vi "MB_TCP_X.vi"(6 "N":i32, 9 "timeouts":T1={"conn_timeout"=1000, "reconn_timeout"=3000, "N attempt max"=3, "t_reset_TTL"=120000, "write_timeout"=10, "read_timeout"=500, "period"=100} {"t_reset_TTL" min=10 max=240000 step=1; "period" min=10 max=100000 step=1; "read_timeout" min=10 max=60000 step=1; "write_timeout" min=1 max=60000 step=1; "N attempt max" min=1 max=5 step=1; "reconn_timeout" min=10 max=240000 step=1; "conn_timeout" min=10 max=240000}, 10 "write enable":bool=TRUE, 11 "stop":bool) -> (0 "error out":errorcluster, 2 "errors":u32, 3 "Z3":u32)   [LabVIEW 2019, in "MB_TCP1.lvlib"]
uses:
  MB_TCP1.lvlib
  Userlib.lvlib
  NI_modbus_upd/NI_modbus_upd.lvlib
  NI_modbus_upd.llb/MB Modbus Command.ctl
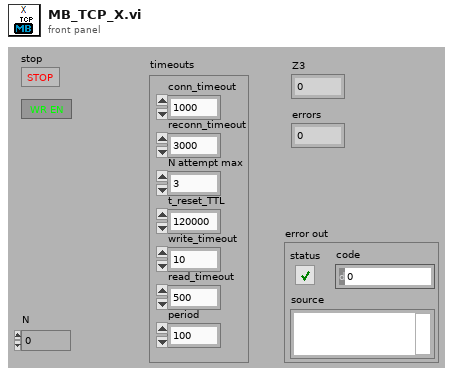
[diagram p1: front panel]
types:
  T1 = cluster{"conn_timeout":i32, "reconn_timeout":u32, "N attempt max":i32, "t_reset_TTL":u32, "write_timeout":i32, "read_timeout":i32, "period":u32}
  T2 = enum16{"Init", "Read", "Read inputs", "Read outputs", "Write", "Write inputs"}
  T3 = enum16{"DI", "DO to write", "DO", "AI", "AO to write", "AO", "DI AI", "DI AO", "DO AI", "DO AO"}
  T4 = enum16{"Start", "Connect", "Write enable", "IP address", "Errors"}
  T5 = typedef "MB Modbus Command.ctl" = cluster{"Function Code":u8, "Starting Address":u16, "Quantity":u16, "Data":u16[], "Discrete":bool[]}
  T6 = cluster{"Transaction ID":u16, "Protocol ID":u16, "Length":u16, "Unit ID":u8}
  T7 = cluster{"Remote IP Address":string, "Remote Port":u16}
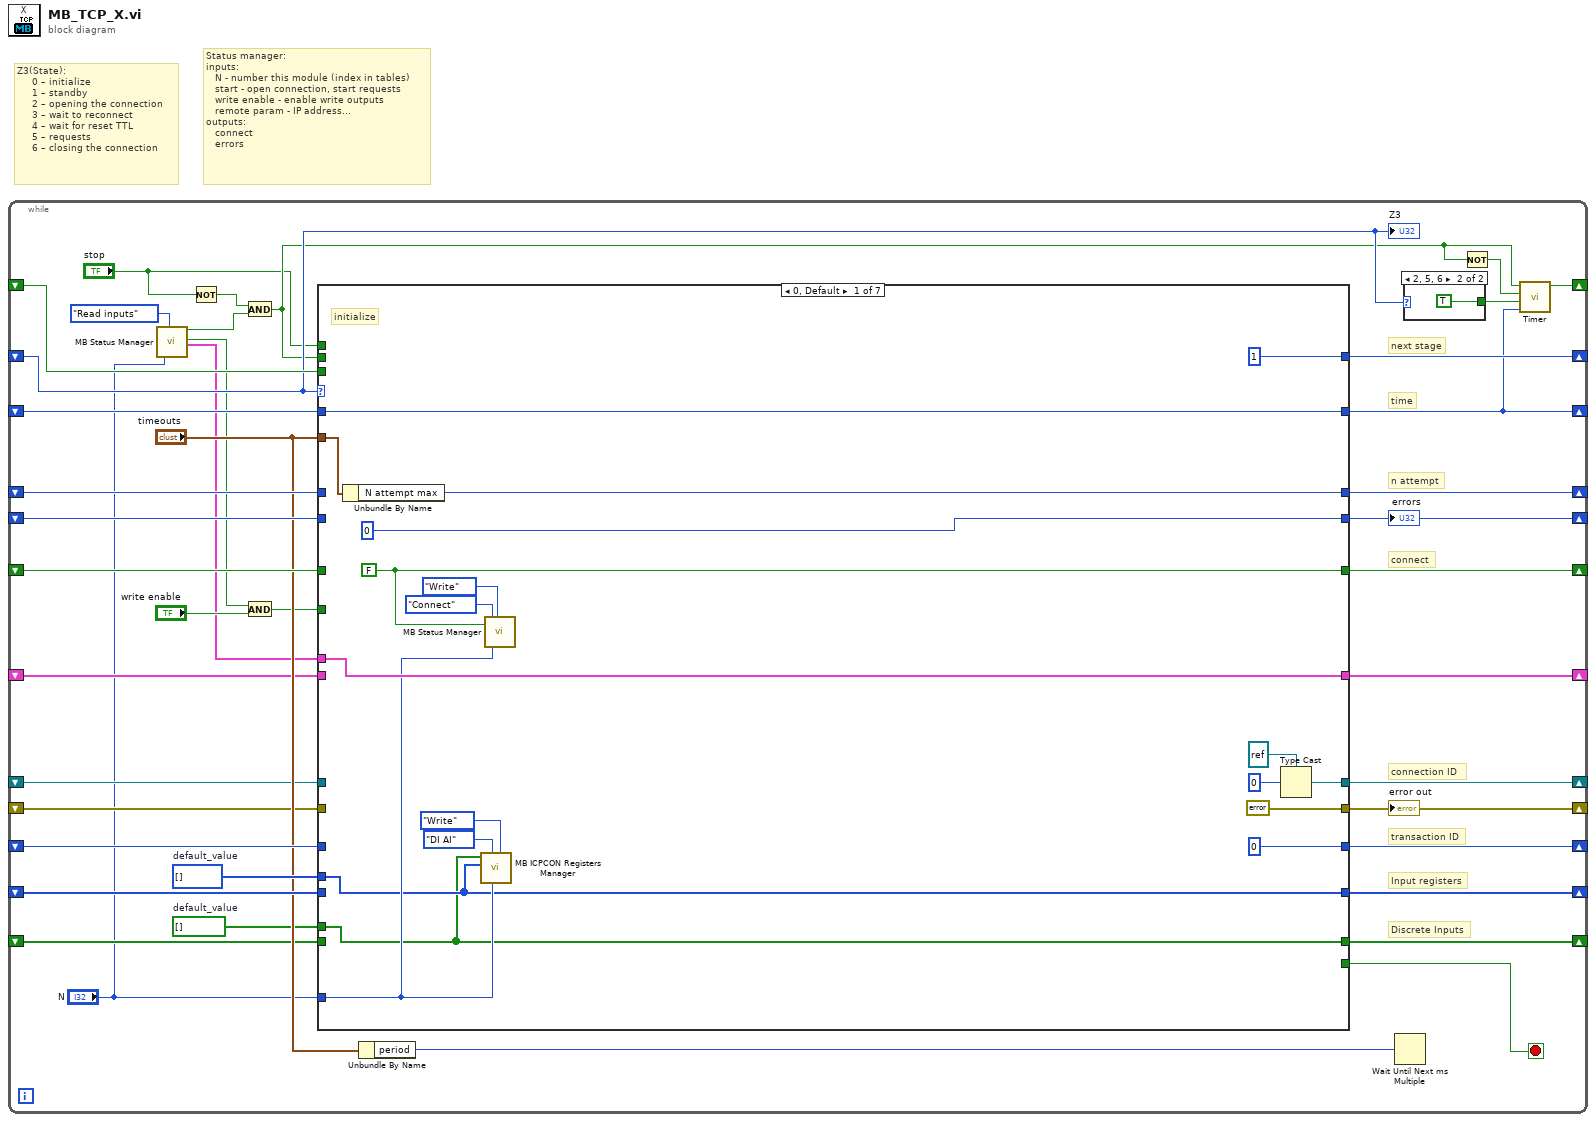
[diagram p0: block diagram]
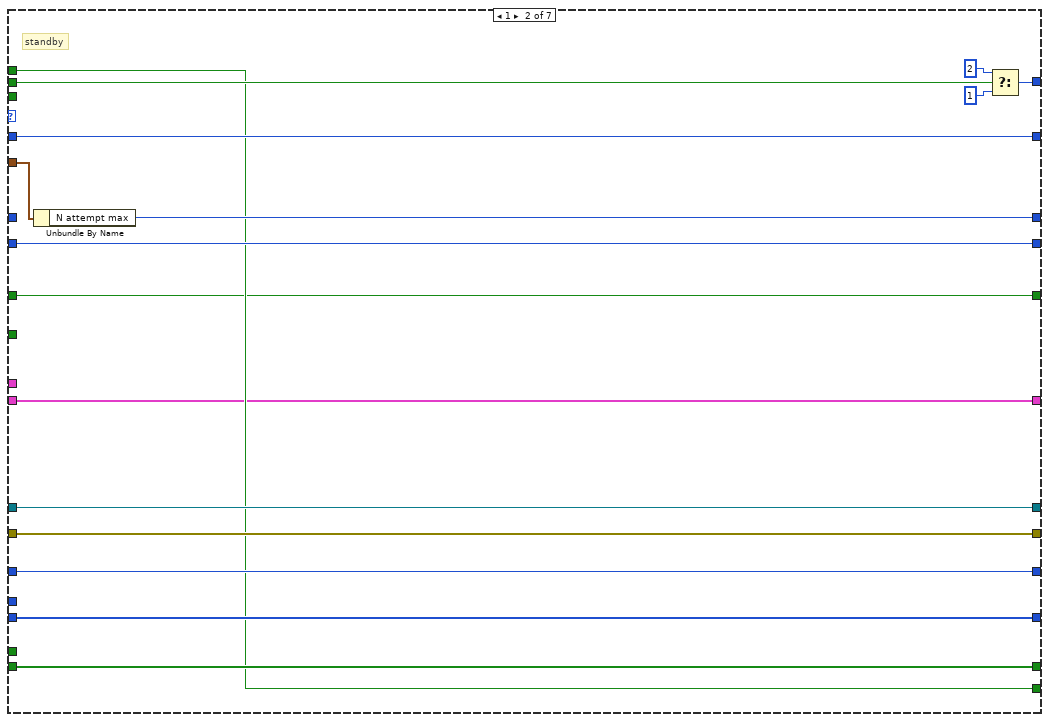
[diagram p2: hidden frame]
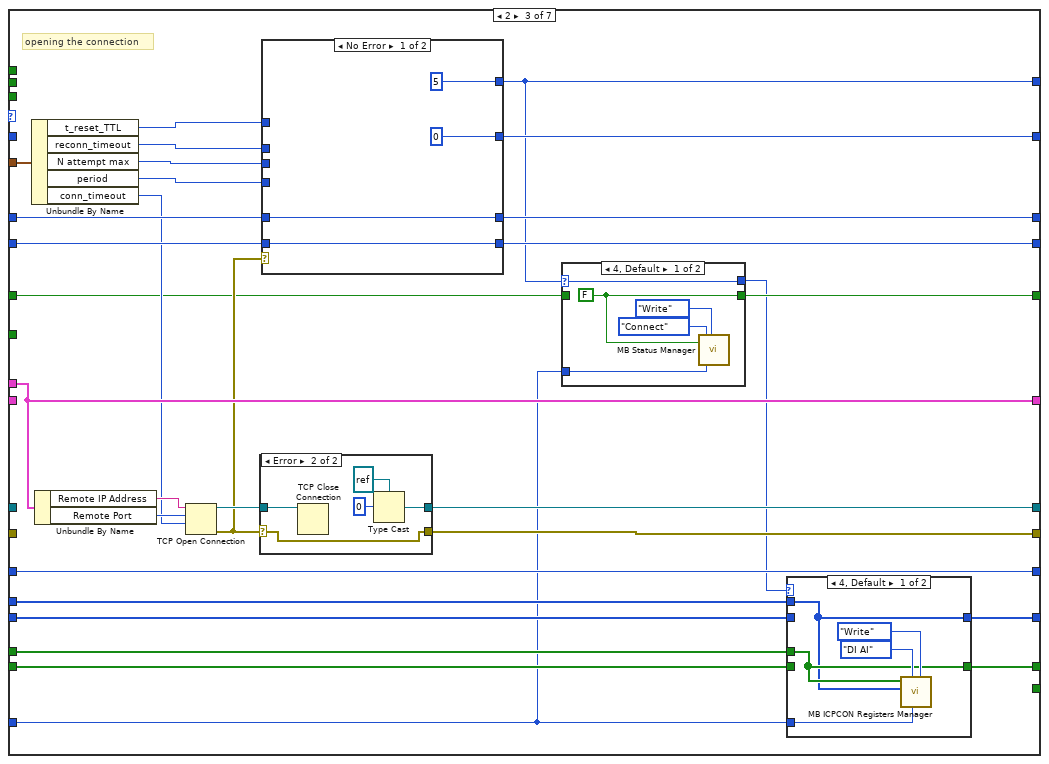
[diagram p3: hidden frame]
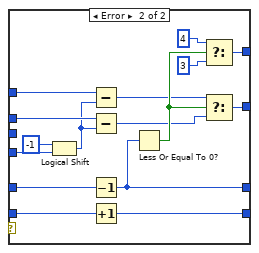
[diagram p7: hidden frame]
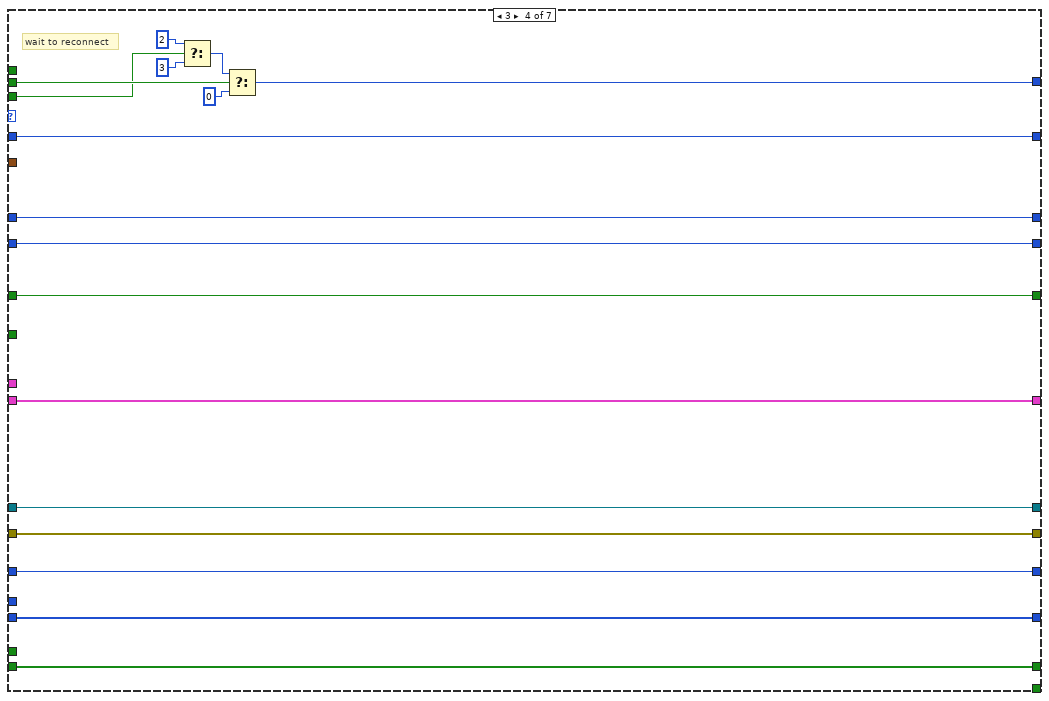
[diagram p8: hidden frame]
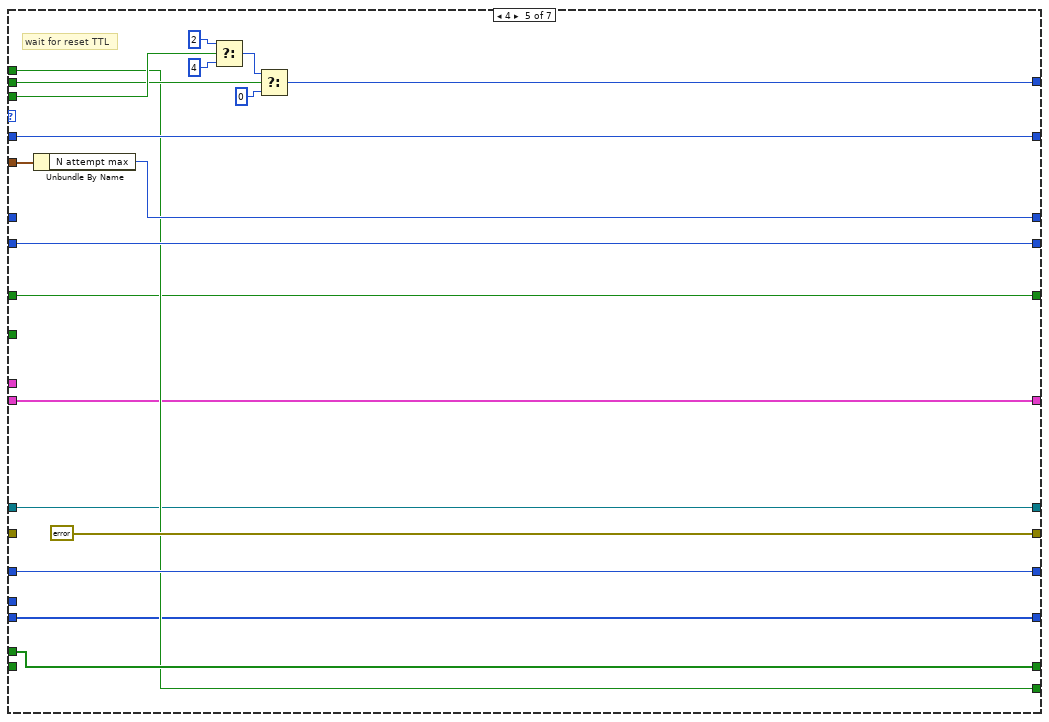
[diagram p9: hidden frame]
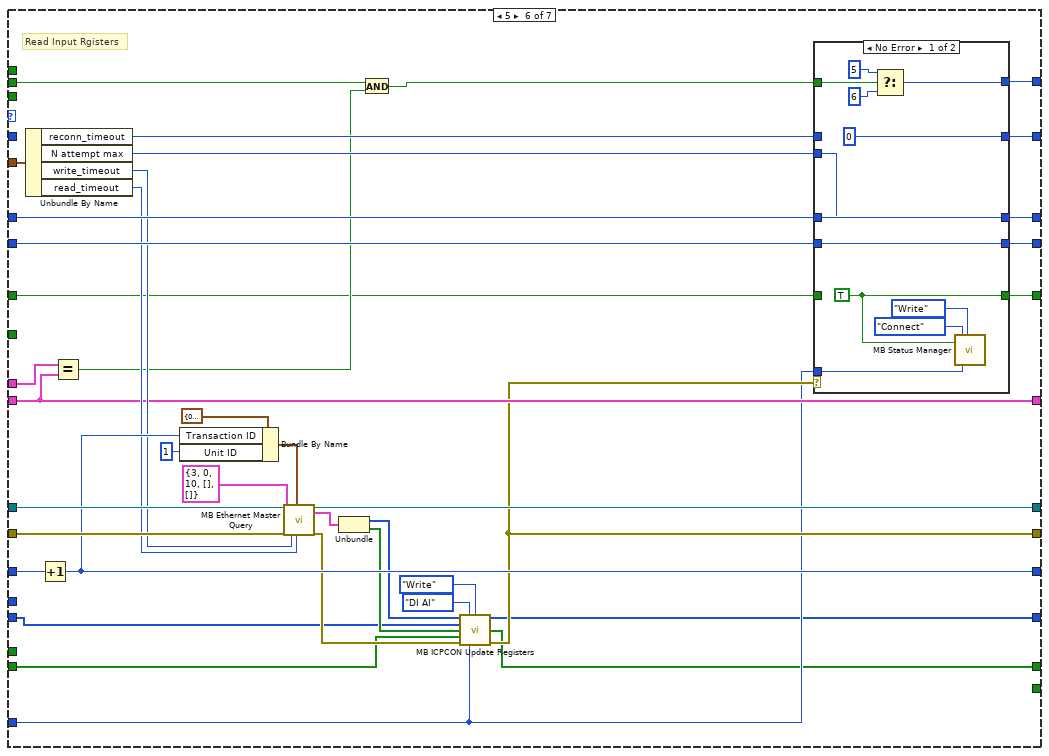
[diagram p10: hidden frame]
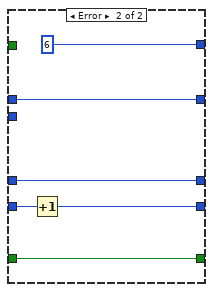
[diagram p11: hidden frame]
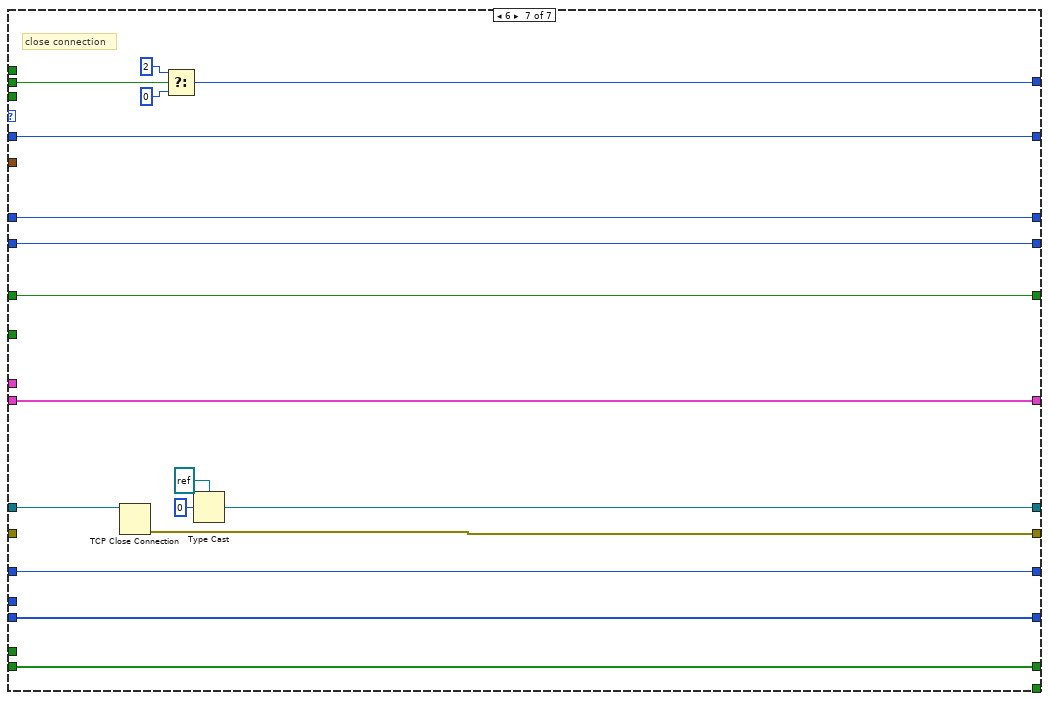
[diagram p12: hidden frame]
diagram:
  # "Status manager:\ninputs:\n   N - number this module (index in tables)\n   start - open connection, start requests\n   write enable - enable write outputs\n   remote param - IP address...\noutputs:\n   connect\n   errors"
  # "Z3(State):\n     0 – initialize \n     1 – standby\n     2 – opening the connection\n     3 – wait to reconnect\n     4 – wait for reset TTL\n     5 – requests\n     6 – closing the connection"
  n1 = while {
    shift-right: [w18] -> _
    shift-left: _ -> [w14]
    shift-right: [w17] -> _
    shift-left: _ -> [w40]
    shift-right: [w39] -> _
    shift-left: _ -> [w37]
    shift-right: [w38] -> _
    shift-left: _ -> [w36]
    shift-right: [w35] -> _
    shift-left: _ -> [w34]
    shift-right: [w33] -> _
    shift-left: _ -> [w19]
    shift-right: [w32] -> _
    shift-left: _ -> [w20]
    shift-right: [w31] -> _
    shift-left: _ -> [w30]
    shift-right: [w29] -> _
    shift-left: _ -> [w28]
    shift-right: [w22] -> _
    shift-left: _ -> [w21]
    shift-right: [w16] -> _
    shift-left: _ -> [w15]
    shift-right: [w7] -> _
    shift-left: _ -> [w6]
    stop <- w10 stop-if-true
    w23 = bool[] []  # default_value
    w27 = u16[] []  # default_value
    # "Discrete Inputs"
    # "Input registers"
    # "connect"
    # "connection ID"
    # "transaction ID"
    # "n attempt"
    # "time"
    # "next stage"
    n2 = call "MB Status Manager.vi"("N"="N", "Function"=T2."Read inputs") -> ("start"=w5:bool, "write enable"=w4:bool, "Remote Param"=w3:T7)  [unwired: 12 in, 3 out]
    n3 = Not(x="stop") -> (.not. x?=w12:bool)
    n4 = And(x=w12, y=w5) -> (x .and. y?=w13:bool)
    n5 = And(x=w4, y="write enable") -> (x .and. y?=w9:bool)
    n6 = case shown="0, Default" w14 {
      tunnel: [w58 w67 w84 w162 w168 w210 w253] -> w33
      tunnel: [errorcluster {"status"=FALSE, "code"=0, "source"=""} ("error out") w66 w82 w161 errorcluster {"status"=FALSE, "code"=0, "source"=""} ("error out") w193 w254] -> w32
      tunnel: w19 -> [_ w67 _ w162 w168 w212 w250]
      tunnel: w20 -> [_ w66 _ w161 _ w211 _]
      tunnel: [w47 w62 w80 w150 w167 w195 w241] -> w35
      tunnel: w34 -> [_ w62 w81 w150 w167 w196 w241]
      tunnel: w3 -> [w50 _ w87 _ _ w202 _]
      tunnel: [w45 w68 w92 w149 w166 w189 w240] -> w29
      tunnel: w28 -> [_ w68 w93 w149 w166 w184 w240]
      tunnel: w30 -> [_ w76 w106 w164 w183 w221 w255]
      tunnel: [u16 0 ("x") w76 w106 w164 w183 w206 w255] -> w31
      tunnel: [w52 w72 w101 w163 w179 w219 w247] -> w39
      tunnel: w37 -> [_ _ w102 w163 _ w219 w247]
      tunnel: [u32 0 ("N attempt max") w75 w104 w160 w182 w218 w252] -> w38
      tunnel: w36 -> [_ w75 w105 w160 w182 w217 w252]
      tunnel: [w54 w74 w98 w159 w181 w214 w251] -> w17
      tunnel: w40 -> [w54 w74 _ w159 w181 _ w251]
      tunnel: "timeouts" -> [w53 w73 w103 _ w180 w220 _]
      tunnel: w13 -> [_ w64 _ w155 w170 w201 w248]
      tunnel: [u32 1 w69 w78 w151 w174 w213 w242] -> w18
      tunnel: w15 -> [_ _ _ w153 w173 _ _]
      tunnel: w27 -> [w45 _ w91 _ _ _ _]
      tunnel: w23 -> [w43 _ w88 _ w171 _ _]
      tunnel: [w43 w65 w89 w152 w171 w188 w245] -> w22
      tunnel: w21 -> [_ w65 w90 w152 _ w187 w245]
      tunnel: "N" -> [w46 _ w79 _ _ w192 _]
      tunnel: "stop" -> [_ w63 _ _ w169 _ _]
      tunnel: [_ w63 _ _ w169 _ _] -> w10
      tunnel: w9 -> [_ _ _ _ _ _ _]
      tunnel: [w50 w61 w87 w148 w165 w199 w239] -> w7
      tunnel: w6 -> [_ w61 _ w148 w165 w199 w239]
      frame 0, Default {
        w47 = FALSE ("connect")
        # "initialize"
        n7 = Unbundle By Name(w53) -> ("N attempt max"=w52:i32)
        n8 = call "MB ICPCON Registers Manager.vi"("Function"=enum16{"Init", "Read", "Write", "Read All"}."Write", "N"=w46, "Table"=T3."DI AI", "Registers In"=w45, "Discrete in"=w43) -> ()  [unwired: 4 in, 3 out]
        n9 = call "MB Status Manager.vi"("connect in"=w47, "Table"=T4."Connect", "N"=w46, "Function"=T2."Write") -> ()  [unwired: 10 in, 6 out]
        n10 = Type Cast(type=refnum<k5> refnum ("connection ID"), x=u32 0) -> (*(type *) &x=w58:refnum<k5>)
      }
      frame 1 {
        # "standby"
        n11 = Unbundle By Name(w73) -> ("N attempt max"=w72:i32)
        n12 = Select(t=u32 2, s=w64, f=u32 1) -> (s? t:f=w69:u32)
      }
      frame 2 {
        # "opening the connection"
        n13 = Unbundle By Name(w103) -> ("t_reset_TTL"=w97:u32, "reconn_timeout"=w99:u32, "N attempt max"=w100:i32, "period"=w94:u32, "conn_timeout"=w86:i32)
        n14 = Unbundle By Name(w87) -> ("Remote IP Address"=w96:string, "Remote Port"=w95:u16)
        n15 = TCP Open Connection(address=w96, remote port or service name=w95, timeout ms (60000)=w86) -> (connection ID=w85:refnum<k5>, error out=w83:errorcluster)  [unwired: 2 in]
        n16 = case shown="Error" w83 {
          selector: w83 -> [w114 w116]
          tunnel: w85 -> [w115 w119]
          tunnel: [w115 w118] -> w84
          tunnel: [w114 w116] -> w82
          frame No Error {
          }
          frame Error {
            n17 = TCP Close Connection(connection ID=w119) -> ()  [unwired: 2 in, 2 out]
            n18 = Type Cast(type=refnum<k5> refnum ("connection ID"), x=u32 0) -> (*(type *) &x=w118:refnum<k5>)
          }
        }
        n19 = case shown="No Error" w83 {
          tunnel: w105 -> [w131 w147]
          tunnel: [w131 w146] -> w104
          tunnel: w102 -> [w130 w145]
          tunnel: [w130 w144] -> w101
          tunnel: w100 -> [_ _]
          tunnel: [u32 5 w141] -> w78
          tunnel: w99 -> [_ w140]
          tunnel: [u32 0 w139] -> w98
          tunnel: w97 -> [_ w136]
          tunnel: w94 -> [_ w134]
          frame No Error {
          }
          frame Error {
            n20 = Logical Shift(y=i16 -1, x=w134) -> (x << y=w132:u32)
            n21 = Subtract(x=w136, y=w132) -> (x-y=w135:u32)
            n22 = Subtract(x=w140, y=w132) -> (x-y=w137:u32)
            n23 = Decrement(x=w145) -> (x-1=w144:i32)
            n24 = Increment(x=w147) -> (x+1=w146:u32)
            n25 = Less Or Equal To 0?(x=w144) -> (x <= 0?=w138:bool)
            n26 = Select(t=u32 4, s=w138, f=u32 3) -> (s? t:f=w141:u32)
            n27 = Select(t=w135, s=w138, f=w137) -> (s? t:f=w139:u32)
          }
        }
        n28 = case shown="4, Default" w78 {
          selector: w78 -> [w108 w112]
          tunnel: w79 -> [w109 _]
          tunnel: [w110 w113] -> w80
          tunnel: w81 -> [_ w113]
          tunnel: [w108 w112] -> w77
          frame 4, Default {
            w110 = FALSE ("f")
            n29 = call "MB Status Manager.vi"("connect in"=w110, "Table"=T4."Connect", "N"=w109, "Function"=T2."Write") -> ()  [unwired: 10 in, 6 out]
          }
          frame 3, 5 {
          }
        }
        n30 = case shown="4, Default" w77 {
          tunnel: w79 -> [w124 _]
          tunnel: [w121 w127] -> w92
          tunnel: w93 -> [_ w127]
          tunnel: w91 -> [w121 _]
          tunnel: w90 -> [_ w126]
          tunnel: [w122 w126] -> w89
          tunnel: w88 -> [w122 _]
          frame 4, Default {
            n31 = call "MB ICPCON Registers Manager.vi"("Function"=enum16{"Init", "Read", "Write", "Read All"}."Write", "N"=w124, "Table"=T3."DI AI", "Registers In"=w121, "Discrete in"=w122) -> ()  [unwired: 4 in, 3 out]
          }
          frame 3, 5 {
          }
        }
      }
      frame 3 {
        # "wait to reconnect"
        n32 = Select(t=u32 2, s=w153, f=u32 3) -> (s? t:f=w154:u32)
        n33 = Select(t=w154, s=w155, f=u32 0) -> (s? t:f=w151:u32)
      }
      frame 4 {
        # "wait for reset TTL"
        n34 = Unbundle By Name(w180) -> ("N attempt max"=w179:i32)
        n35 = Select(t=u32 2, s=w173, f=u32 4) -> (s? t:f=w175:u32)
        n36 = Select(t=w175, s=w170, f=u32 0) -> (s? t:f=w174:u32)
      }
      frame 5 {
        # "Read Input Rgisters"
        n37 = Unbundle By Name(w220) -> ("reconn_timeout"=w215:u32, "N attempt max"=w216:i32, "write_timeout"=w204:i32, "read_timeout"=w203:i32)
        n38 = Increment(x=w221) -> (x+1=w206:u16)
        n39 = Equal?(x=w202, y=w199) -> (x = y?=w198:bool)
        n40 = Bundle By Name(cluster=T6 {"Transaction ID"=0, "Protocol ID"=0, "Length"=0, "Unit ID"=0} ("MBAP Header"), "Transaction ID"=w206, "Unit ID"=u8 1) -> (w205:T6)
        n41 = call "MB Ethernet Master Query.vi"("TCP Connection Refnum in"=w212, "Modbus Command"=T5 {"Function Code"=3, "Starting Address"=0, "Quantity"=10, "Data"=[], "Discrete"=[]}, "error in (no error)"=w211, "Write Timeout"=w204, "MBAP Header"=w205, "Read Timeout"=w203) -> ("TCP Connection Refnum (dup)"=w210:refnum<k5>, "Registers"=w209:cluster{"Registers":u16[], "Discrete":bool[]}, "error out"=w194:errorcluster)  [unwired: 9 in, 2 out]
        n42 = Unbundle(w209) -> ("Registers"=w185:u16[], "Discrete"=w186:bool[])
        n43 = And(x=w201, y=w198) -> (x .and. y?=w200:bool)
        n44 = call "MB ICPCON Update Registers.vi"("Registers In"=w185, "Table"=T3."DI AI", "Function"=enum16{"Init", "Read", "Write", "Read All"}."Write", "Default Registers In"=w184, "Discrete in"=w186, "Default Discrete in"=w187, "error in (no error)"=w194, "N"=w192) -> ("Registers"=w189:u16[], "Discretes"=w188:bool[], "error out"=w193:errorcluster)  [unwired: 5 in]
        n45 = case shown="No Error" w193 {
          tunnel: w217 -> [w226 w238]
          tunnel: [w226 w237] -> w218
          tunnel: [w228 u32 6] -> w213
          tunnel: w219 -> [_ w235]
          tunnel: w216 -> [w232 _]
          tunnel: [w232 w235] -> _
          tunnel: w215 -> [_ w234]
          tunnel: [u32 0 w234] -> w214
          tunnel: w200 -> [w227 _]
          tunnel: w196 -> [_ w233]
          tunnel: [w224 w233] -> w195
          tunnel: w192 -> [w223 _]
          frame No Error {
            w224 = TRUE ("f")
            n46 = Select(t=u32 5, s=w227, f=u32 6) -> (s? t:f=w228:u32)
            n47 = call "MB Status Manager.vi"("connect in"=w224, "Table"=T4."Connect", "N"=w223, "Function"=T2."Write") -> ()  [unwired: 10 in, 6 out]
          }
          frame Error {
            n48 = Increment(x=w238) -> (x+1=w237:u32)
          }
        }
      }
      frame 6 {
        # "close connection"
        n49 = TCP Close Connection(connection ID=w250) -> (error out=w254:errorcluster)  [unwired: 2 in, 1 out]
        n50 = Select(t=u32 2, s=w248, f=u32 0) -> (s? t:f=w242:u32)
        n51 = Type Cast(type=refnum<k5> refnum ("connection ID"), x=u32 0) -> (*(type *) &x=w253:refnum<k5>)
      }
    }
    "error out" <- w32
    "errors" <- w38
    n52 = Unbundle By Name("timeouts") -> ("period"=w25:u32)
    n53 = Wait Until Next ms Multiple(millisecond multiple=w25) -> ()  [unwired: 1 out]
    n54 = case shown="2, 5, 6" w14 {
      tunnel: [_ TRUE] -> w24
      frame 0, Default {
      }
      frame 2, 5, 6 {
      }
    }
    n55 = Not(x=w13) -> (.not. x?=w41:bool)
    n56 = call "Timer.vi"("ms"=w17, "Load (F)"=w24, "Reset (F)"=w41, "Start (T)"=w13) -> ("End"=w16:bool)  [unwired: 5 in, 1 out]
    "Z3" <- w14
  }
